vi "CRYGet Difference Array.vi"(4 "String2":string[](array[string]), 6 "String1":string[](array[string]), 8 "sOption":string, 9 "Array 2":i32[](array[numeric]), 11 "Array 1":i32[](array[numeric])) -> (1 "StringDiff Out":string[](array[string]), 3 "Diff Out":i32[](array[numeric]))   [LabVIEW 2013]
panel:
  # "-"
  # "="
  # "-"
  # "="
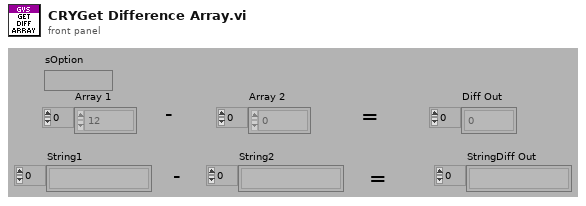
[diagram p1: front panel]
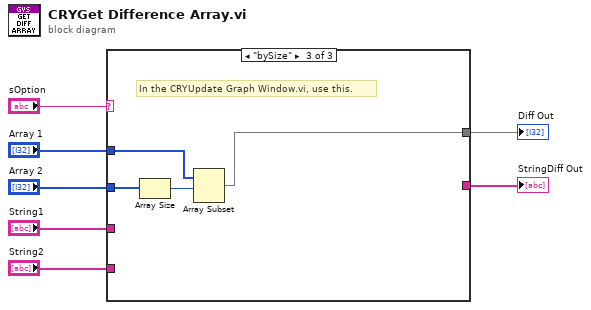
[diagram p0: block diagram]
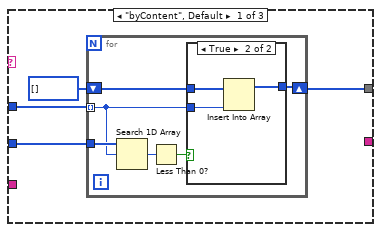
[diagram p2: hidden frame]
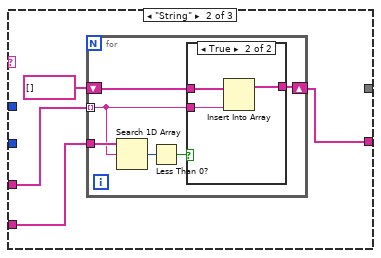
[diagram p4: hidden frame]
diagram:
  n1 = case shown="\"bySize\"" "sOption" {
    tunnel: [w10 _ w36] -> w7
    tunnel: "Array 2" -> [w9 _ w39]
    tunnel: "Array 1" -> [w8 _ w38]
    tunnel: "String1" -> [_ w24 _]
    tunnel: "String2" -> [_ w23 _]
    tunnel: [_ w22 _] -> w1
    frame "byContent", Default {
      n2 = for {
        shift-right: [w13] -> w10
        shift-left: i32[] [] ("Value") -> [w14]
        tunnel: w8 -> [w12] mode=indexing
        tunnel: w9 -> [w16]
        n3 = Search 1D Array(1D array=w16, element=w12) -> (index of element=w17:i32)  [unwired: 1 out]
        n4 = Less Than 0?(x=w17) -> (x < 0?=w15:bool)
        n5 = case shown="True" w15 {
          tunnel: w12 -> [_ w21]
          tunnel: w14 -> [w18 w20]
          tunnel: [w18 w19] -> w13
          frame False {
          }
          frame True {
            n6 = Insert Into Array(array=w20, new element=w21) -> (w19:i32[])  [unwired: 1 in]
          }
        }
      }
    }
    frame "String" {
      n7 = for {
        shift-right: [w27] -> w22
        shift-left: string[] [] ("String1") -> [w28]
        tunnel: w24 -> [w26] mode=indexing
        tunnel: w23 -> [w30]
        n8 = Search 1D Array(1D array=w30, element=w26) -> (index of element=w31:i32)  [unwired: 1 out]
        n9 = Less Than 0?(x=w31) -> (x < 0?=w29:bool)
        n10 = case shown="True" w29 {
          tunnel: w26 -> [_ w35]
          tunnel: w28 -> [w32 w34]
          tunnel: [w32 w33] -> w27
          frame False {
          }
          frame True {
            n11 = Insert Into Array(array=w34, new element=w35) -> (w33:string[])  [unwired: 1 in]
          }
        }
      }
    }
    frame "bySize" {
      # "In the CRYUpdate Graph Window.vi, use this."
      n12 = Array Size(array=w39) -> (size(s)=w37:i32)
      n13 = Array Subset(array=w38, index=w37) -> (w36:i32[])  [unwired: 1 in]
    }
  }
  "Diff Out" <- w7
  "StringDiff Out" <- w1
